vi "isStaticScan.vi"(11 "Move Type":T1) -> (3 "Boolean":bool)   [LabVIEW 2012]
uses:
  typedefs/Move Type.ctl
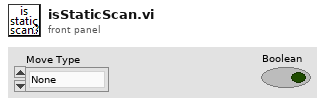
[diagram p1: front panel]
types:
  T1 = typedef "Move Type.ctl" = enum16{"None", "Continuous", "Discrete"}
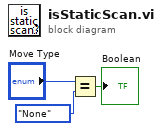
[diagram p0: block diagram]
diagram:
  n1 = Equal?(x="Move Type", y=Move_Type."None") -> (x = y?=→"Boolean":bool)
